vi "measure.vi"(8 "error in (no error)":errorcluster, 11 "DmmNiPxi in":refnum<class "DmmNi.lvclass">) -> (0 "error out":errorcluster, 2 "value":dbl, 3 "DmmNiPxi out":refnum<class "DmmNi.lvclass">)   [LabVIEW 2023, in "DmmNi.lvclass"]
doc: "<b>Author:</b> Wolfgang\n<b>Description:</b> initiate a measurement on Dmm and return result"
uses:
  DmmNi.lvclass
  DmmNi.lvclass/DmmNi.ctl
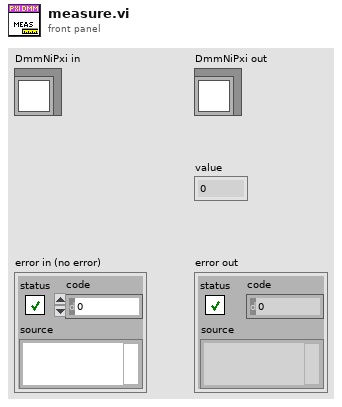
[diagram p1: front panel]
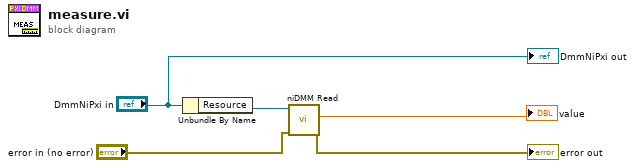
[diagram p0: block diagram]
diagram:
  n1 = Unbundle By Name("DmmNiPxi in") -> ("Resource"=w5:refnum<k15>)
  n2 = call <instrlib>:"niDMM Read.vi"("error in (no error)"="error in (no error)", "instrument handle"=w5) -> ("error out"=→"error out":errorcluster, "Measurement"=→"value":dbl)  [unwired: 7 in, 1 out]
  "DmmNiPxi out" <- "DmmNiPxi in"
